vi "SV TDMS Write Even-Angle Signal (N Ch).vi"(0 "tdms file":refnum<k34>, 1 "write channel properties":bool=TRUE, 5 "group name in":string="Even-Angle_Signal", 7 "channel names in":string[](array[string]), 9 "even-angle signals":cluster{"r0":dbl, "dr":dbl, "Y":dbl[]}[](array[cluster]) {"r0" format="%.2p"; "dr" format="%.2p"; "Y" format="%.2f"}, 11 "error in":errorcluster, 12 "even-angle channel info":T2[](array[typedef]) {"channel info"."pregain" format="%.2f"; "channel info"."weighting filter" items=["Linear", "A-weighting", "B-weighting", "C-weighting", "ITU-R 468-4", "Dolby", "CCITT", "C-message", "Wb", "Wc", "Wd", "We", "Wf", "Wh", "Wj", "Wk", "Wm", "AES17 20 kHz lowpass", "AES17 40 kHz lowpass", "AES17 20 kHz highpass", "AES17 40 kHz highpass"]; "channel info"."dB reference" format="%^.1e"; "channel info"."engineering units" items=["custom..."=0, "V"=1, "A"=21, "C"=30, "pC"=31, "s"=32, "-"=29, "Pa"=2, "N"=20, "g"=3, "m/s^2"=4, "m/s"=5, "m"=6, "mm/s"=12, "mm"=13, "micron/s"=14, "micron"=15, "in/s^2"=7, "in/s"=8, "in"=9, "mil/s"=10, "mil"=11, "rad/s^2"=16, "rad/s"=17, "rad"=18, "deg/s^2"=26, "deg/s"=27, "deg"=28, "RPM"=22, "cycle/s^2"=23, "Hz"=24, "cycle"=25, "strain"=19]; "channel info"."sensor sensitivity" format="%#_5f"}, 13 "even-angle position info":T1) -> (4 "tdms file out":refnum<k34>, 6 "group name out":string, 8 "channel names out":string[](array[string]), 15 "error out":errorcluster)   [LabVIEW 2017]
doc: "Writes data to the specified .tdms file in a format specific to the polymorphic instance. Wire data to the <B>scaled signal [EU]</B> input to determine the polymorphic instance to use or manually select the instance."
uses:
  <vilib>/addons/_NISVFA/_Shared subVIs/Controls/svc_Resampled Channel Info.ctl
  <vilib>/addons/_NISVFA/_Shared subVIs/Controls/svc_Channel Info.ctl
  <vilib>/addons/_NISVFA/_Shared subVIs/Controls/svc_Engineering Units Text Ring.ctl
  <vilib>/addons/_NISVFA/_Shared subVIs/Controls/svc_Weighting Filter Text Ring.ctl
  <vilib>/addons/_NISVFA/_Shared subVIs/Controls/svc_Position Info.ctl
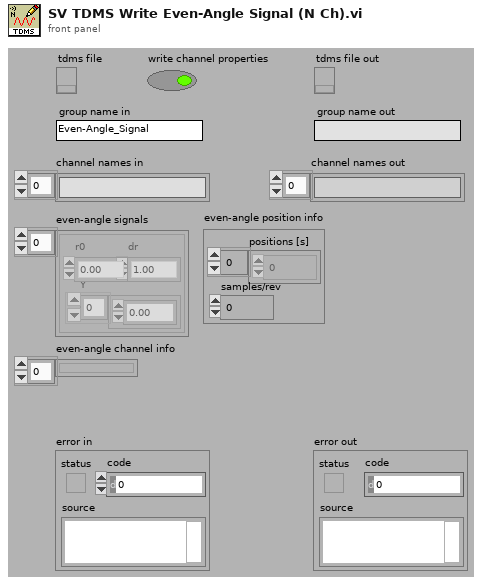
[diagram p1: front panel]
types:
  T1 = typedef "svc_Position Info.ctl" = cluster{"positions [s]":dbl[], "samples/rev":dbl}
  T2 = typedef "svc_Resampled Channel Info.ctl" = cluster{"channel name":string, "description":string, " channel info":T3}
  T3 = typedef "svc_Channel Info.ctl" = cluster{"sensor sensitivity":dbl, "engineering units":T4, "dB reference":dbl, "custom label":string, "weighting filter":T5, "pregain":dbl}
  T4 = typedef "svc_Engineering Units Text Ring.ctl" = u16
  T5 = typedef "svc_Weighting Filter Text Ring.ctl" = u16
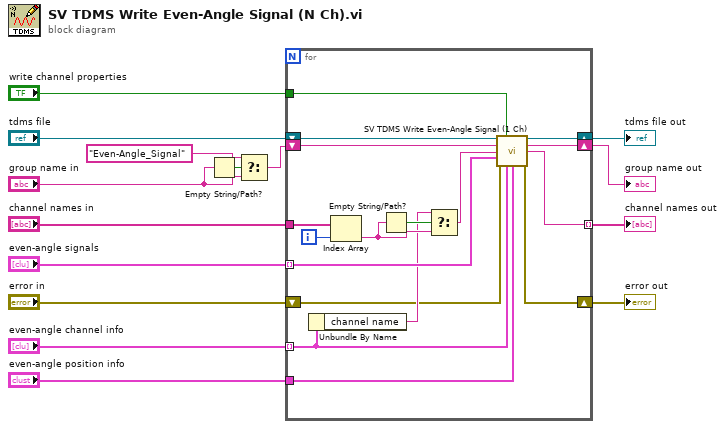
[diagram p0: block diagram]
diagram:
  n1 = Empty String/Path?(string/path="group name in") -> (empty?=w8:bool)
  n2 = Select(t="Even-Angle_Signal", s=w8, f="group name in") -> (s? t:f=w6:string)
  n3 = for {
    tunnel: "channel names in" -> [w30]
    tunnel: "even-angle channel info" -> [w21] mode=indexing
    tunnel: "even-angle signals" -> [w25] mode=indexing
    tunnel: [w22] -> w9 mode=indexing
    shift-right: [w24] -> w12
    shift-left: "tdms file" -> [w27]
    shift-right: [w18] -> w13
    shift-left: "error in" -> [w19]
    shift-right: [w23] -> w10
    shift-left: w6 -> [w28]
    tunnel: "write channel properties" -> [w17]
    tunnel: "even-angle position info" -> [w16]
    i -> [w31]
    n4 = Unbundle By Name(w21) -> ("channel name"=w20:string)
    n5 = Index Array(array=w30, index=w31) -> (element=w29:string)
    n6 = Empty String/Path?(string/path=w29) -> (empty?=w32:bool)
    n7 = Select(t=w20, s=w32, f=w29) -> (s? t:f=w26:string)
    n8 = call <vilib>:"SV TDMS Write Even-Angle Signal (1 Ch).vi"("tdms file"=w27, "write channel properties"=w17, "group name in"=w28, "channel name in"=w26, "even-angle signal"=w25, "error in"=w19, "even-angle channel info"=w21, "even-angle position info"=w16) -> ("tdms file out"=w24:refnum<k34>, "group name out"=w23:string, "channel name out"=w22:string, "error out"=w18:errorcluster)  [unwired: 4 in]
  }
  "error out" <- w13
  "tdms file out" <- w12
  "group name out" <- w10
  "channel names out" <- w9
